vi "check_pixelfly_status.vi"() -> ()   [LabVIEW 2013]
panel:
  out "PixelFly in Use?":bool
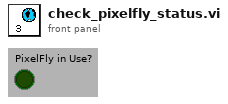
[diagram p1: front panel]
diagram:
